vi "数据拼接.vi"() -> ()   [LabVIEW 2012]
panel:
  out "x+y":dbl format="%#.3g"
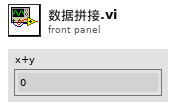
[diagram p1: front panel]
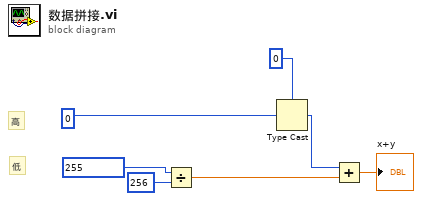
[diagram p0: block diagram]
diagram:
  # "低"
  # "高"
  n1 = Divide(x=u8 255, y=u16 256) -> (x/y=w2:dbl)
  n2 = Type Cast(type=i8 0, x=u8 0) -> (*(type *) &x=w3:i8)
  n3 = Add(x=w3, y=w2) -> (x+y=→"x+y":dbl)
